vi "Init_Tracks&Coord-1.vi"() -> (0 "Tracks, coordinates":T1)   [LabVIEW 2013]
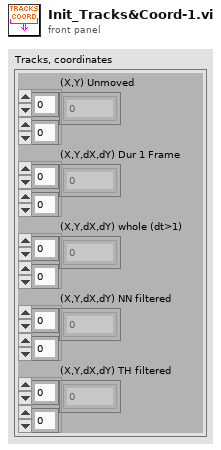
[diagram p1: front panel]
types:
  T1 = cluster{"(X,Y) Unmoved":dbl[][], "(X,Y,dX,dY) Dur 1 Frame":dbl[][], "(X,Y,dX,dY) whole (dt>1)":dbl[][], "(X,Y,dX,dY) NN filtered":dbl[][], "(X,Y,dX,dY) TH filtered":dbl[][]}
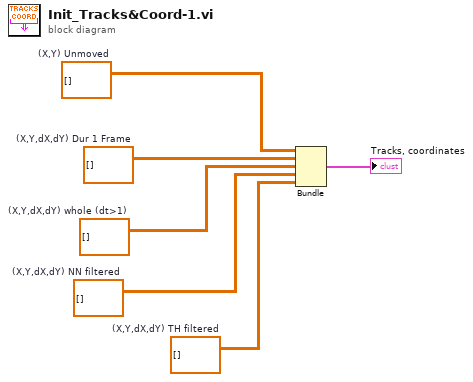
[diagram p0: block diagram]
diagram:
  w3 = dbl[][] []  # (X,Y,dX,dY) TH filtered
  w2 = dbl[][] []  # (X,Y,dX,dY) NN filtered
  w5 = dbl[][] []  # (X,Y,dX,dY) Dur 1 Frame
  w6 = dbl[][] []  # (X,Y) Unmoved
  w4 = dbl[][] []  # (X,Y,dX,dY) whole (dt>1)
  n1 = Bundle("(X,Y) Unmoved"=w6, "(X,Y,dX,dY) Dur 1 Frame"=w5, "(X,Y,dX,dY) whole (dt>1)"=w4, "(X,Y,dX,dY) NN filtered"=w2, "(X,Y,dX,dY) TH filtered"=w3) -> (→"Tracks, coordinates":T1)  [unwired: 1 in]
